vi "AVS_GetIpConfig.vi"(2 "a_Data":u8[](array[numeric]), 3 "a_hDevice":i32) -> (0 "a_Data":u8[](array[numeric]), 1 "Output Value":i32)   [LabVIEW 2018]
uses:
  avaspecx64.dll
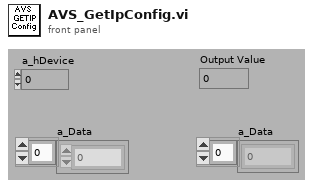
[diagram p1: front panel]
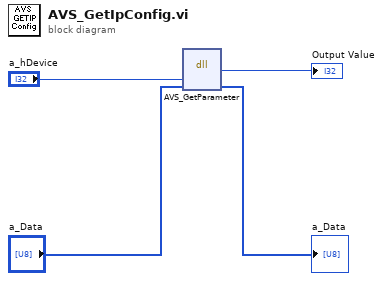
[diagram p0: block diagram]
diagram:
  n1 = dll-call lib="C:/AvaSpecX64-DLL_9.7/examples/LabView/LabViewSingleChan/avaspecx64.dll" fn="AVS_GetParameter"("a_hDevice"="a_hDevice", "a_Data"="a_Data") -> ("return type"=→"Output Value":i32, "a_Data"=→"a_Data":u8[])  [unwired: 4 in, 2 out]
